vi "AddDUTRef.vi"(10 "GuiRef输入":T1, 11 "Controls[]":refnum<vi>[](array[refnum])) -> (3 "GuiRef输出":T1)   [LabVIEW 2013]
uses:
  SystemCode/SysControl/Reference.ctl
  SystemCode/SysControl/TestItemsCTL.ctl
  SystemCode/SysControl/Slot.ctl
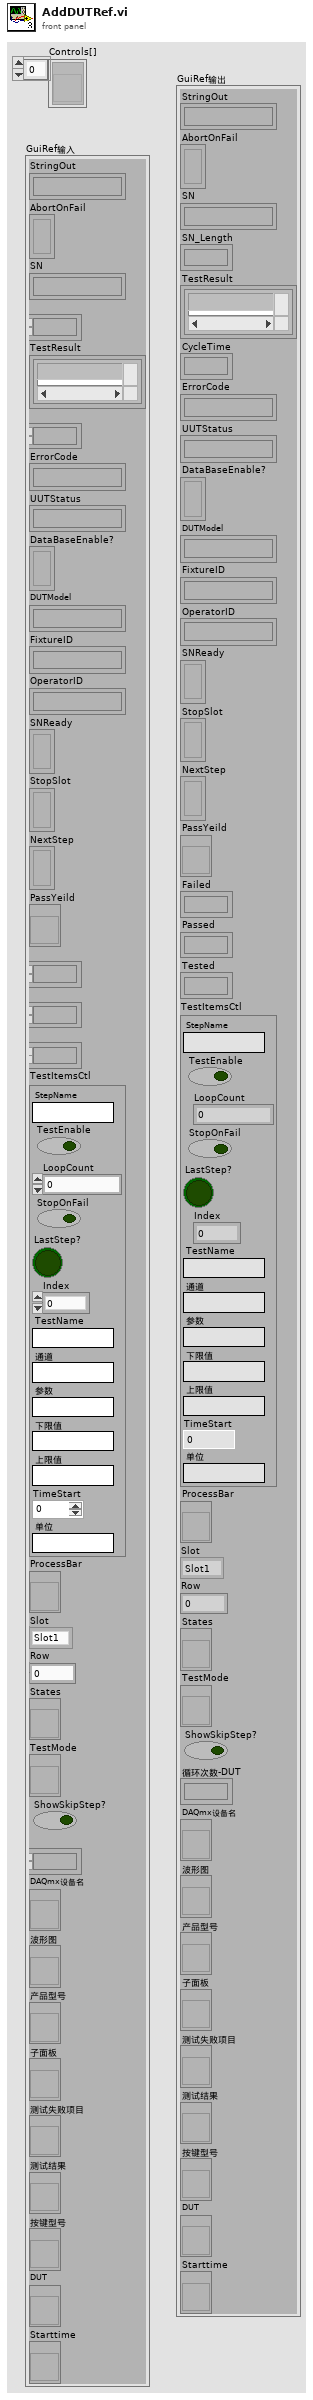
[diagram p1: front panel]
types:
  T1 = typedef "Reference.ctl" = cluster{"StringOut":refnum<vi>, "AbortOnFail":refnum<vi>, "SN":refnum<vi>, "SN_Length":refnum<vi>, "TestResult":refnum<vi>, "CycleTime":refnum<vi>, "ErrorCode":refnum<vi>, "UUTStatus":refnum<vi>, "DataBaseEnable?":refnum<vi>, "DUTModel":refnum<vi>, "FixtureID":refnum<vi>, "OperatorID":refnum<vi>, "SNReady":refnum<vi>, "StopSlot":refnum<vi>, "NextStep":refnum<vi>, "PassYeild":refnum<vi>, "Failed":refnum<vi>, "Passed":refnum<vi>, "Tested":refnum<vi>, "TestItemsCtl":T2, "ProcessBar":refnum<vi>, "Slot":T3, "Row":i32, "States":refnum<vi>, "TestMode":refnum<vi>, "ShowSkipStep?":bool, "循环次数-DUT":refnum<vi>, "DAQmx设备名":refnum<vi>, "波形图":refnum<vi>, "产品型号":refnum<vi>, "子面板":refnum<vi>, "测试失败项目":refnum<vi>, "测试结果":refnum<vi>, "按键型号":refnum<vi>, "DUT":refnum<vi>, "Starttime":refnum<vi>}
  T2 = typedef "TestItemsCTL.ctl" = cluster{"StepName":string, "TestEnable":bool, "LoopCount":i32, "StopOnFail":bool, "LastStep?":bool, "Index":i32, "TestName":string, "通道":string, "参数":string, "下限值":string, "上限值":string, "TimeStart":u32, "单位":string}
  T3 = typedef "Slot.ctl" = enum16{"Slot1", "Slot2", "Slot3", "Slot4"}
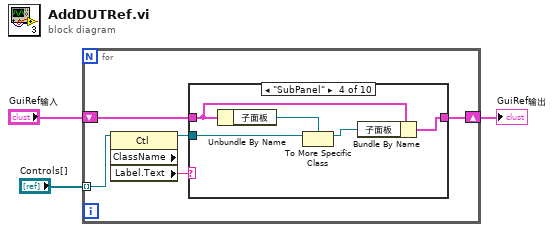
[diagram p0: block diagram]
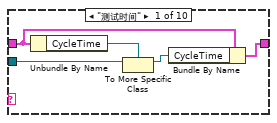
[diagram p2: hidden frame]
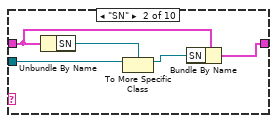
[diagram p3: hidden frame]
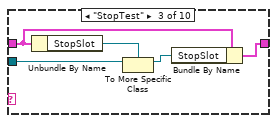
[diagram p4: hidden frame]
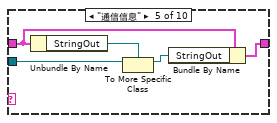
[diagram p5: hidden frame]
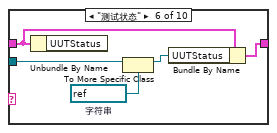
[diagram p6: hidden frame]
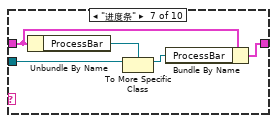
[diagram p7: hidden frame]
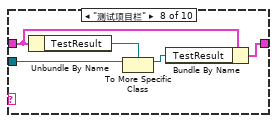
[diagram p8: hidden frame]
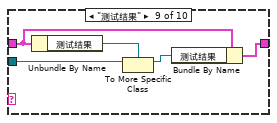
[diagram p9: hidden frame]
diagram:
  n1 = for {
    tunnel: "Controls[]" -> [w8] mode=indexing
    shift-right: [w4] -> w1
    shift-left: "GuiRef输入" -> [w5]
    n2 = property class="Ctl" props=["ClassName", "Label", "Text"](reference=w8) -> (reference out=w7:refnum<vi>, "Label.Text"=w6:string)  [unwired: 1 in, 2 out]
    n3 = case shown="\"SubPanel\"" w6 {
      tunnel: w7 -> [w13 w18 w23 w28 w33 w38 w43 w48 w53 _]
      tunnel: w5 -> [w10 w15 w21 w26 w30 w35 w40 w45 w50 w54]
      tunnel: [w11 w16 w22 w27 w31 w36 w41 w46 w51 w54] -> w4
      frame "测试时间" {
        n4 = Unbundle By Name(w10) -> ("CycleTime"=w9:refnum<vi>)
        n5 = To More Specific Class(target class=w9, reference=w13) -> (specific class reference=w12:refnum<vi>)  [unwired: 1 in, 1 out]
        n6 = Bundle By Name(cluster=w10, "CycleTime"=w12) -> (w11:T1)
      }
      frame "SN" {
        n7 = Unbundle By Name(w15) -> ("SN"=w14:refnum<vi>)
        n8 = To More Specific Class(target class=w14, reference=w18) -> (specific class reference=w17:refnum<vi>)  [unwired: 1 in, 1 out]
        n9 = Bundle By Name(cluster=w15, "SN"=w17) -> (w16:T1)
      }
      frame "StopTest" {
        n10 = Unbundle By Name(w21) -> ("StopSlot"=w20:refnum<vi>)
        n11 = To More Specific Class(target class=w20, reference=w23) -> (specific class reference=w19:refnum<vi>)  [unwired: 1 in, 1 out]
        n12 = Bundle By Name(cluster=w21, "StopSlot"=w19) -> (w22:T1)
      }
      frame "SubPanel" {
        n13 = Unbundle By Name(w26) -> ("子面板"=w25:refnum<vi>)
        n14 = To More Specific Class(target class=w25, reference=w28) -> (specific class reference=w24:refnum<vi>)  [unwired: 1 in, 1 out]
        n15 = Bundle By Name(cluster=w26, "子面板"=w24) -> (w27:T1)
      }
      frame "通信信息" {
        n16 = Unbundle By Name(w30) -> ("StringOut"=w29:refnum<vi>)
        n17 = To More Specific Class(target class=w29, reference=w33) -> (specific class reference=w32:refnum<vi>)  [unwired: 1 in, 1 out]
        n18 = Bundle By Name(cluster=w30, "StringOut"=w32) -> (w31:T1)
      }
      frame "测试状态" {
        w34 = refnum<vi> refnum  # 字符串
        n19 = Unbundle By Name(w35) -> ()  [unwired: 1 out]
        n20 = To More Specific Class(target class=w34, reference=w38) -> (specific class reference=w37:refnum<vi>)  [unwired: 1 in, 1 out]
        n21 = Bundle By Name(cluster=w35, "UUTStatus"=w37) -> (w36:T1)
      }
      frame "进度条" {
        n22 = Unbundle By Name(w40) -> ("ProcessBar"=w39:refnum<vi>)
        n23 = To More Specific Class(target class=w39, reference=w43) -> (specific class reference=w42:refnum<vi>)  [unwired: 1 in, 1 out]
        n24 = Bundle By Name(cluster=w40, "ProcessBar"=w42) -> (w41:T1)
      }
      frame "测试项目栏" {
        n25 = Unbundle By Name(w45) -> ("TestResult"=w44:refnum<vi>)
        n26 = To More Specific Class(target class=w44, reference=w48) -> (specific class reference=w47:refnum<vi>)  [unwired: 1 in, 1 out]
        n27 = Bundle By Name(cluster=w45, "TestResult"=w47) -> (w46:T1)
      }
      frame "测试结果" {
        n28 = Unbundle By Name(w50) -> ("测试结果"=w49:refnum<vi>)
        n29 = To More Specific Class(target class=w49, reference=w53) -> (specific class reference=w52:refnum<vi>)  [unwired: 1 in, 1 out]
        n30 = Bundle By Name(cluster=w50, "测试结果"=w52) -> (w51:T1)
      }
      frame Default {
      }
    }
  }
  "GuiRef输出" <- w1
